vi "AlliGator Run Source Image Python Function.vi"(8 "error in (no error)":errorcluster, 9 "Source Image":T5, 10 "Python Function Info":T1={"Script Path"=path "", "Function Name"="", "Function Parent Menu"="", "API Version"="", "Function Input Parameters"=[], "Function Outputs"=[], "Function Doc String"="", "Function Display Name"="", "Function Target Type"=enum."Window Menu", "Function Target Window"="", "Parent Menu Location"="", "Item Menu Tag"="", "Is preceded by Separator"=FALSE}, 11 "Data Value Reference in":refnum<data-value>) -> (0 "error out":errorcluster, 1 "Message":string, 2 "Function Output Type":string, 3 "Data Value Reference out":refnum<data-value>)   [LabVIEW 2021, in "AlliGator Python Plugins.lvlib"]
doc: "Runs image-related python function."
uses:
  AlliGator Python Plugins.lvlib
  Internal Variables/AlliGator Internal Variables v2.ctl
  <vilib>/vision/Image Controls.llb/IMAQ Image.ctl
  Internal Variables/AlliGator Gate Image Set.ctl
  Files/AlliGator FLI Dataset Type.ctl
  Files/AlliGator Data Series Type.ctl
  Dual-Channel Datasets/AlliGator Dataset Channel.ctl
  Settings/AlliGator Gate Arithmetic.ctl
  Source Image/AlliGator Displayed Image.ctl
  Image/Named ROI Description.ctl
  Phasor Graph/AlliGator Decay Metadata v3.ctl
  Decay Analysis/Decay Preprocessing/AlliGator Decay Background Subtraction Info.ctl
  Decay Analysis/Decay Preprocessing/AlliGator Baseline Subtraction Method.ctl
  Graphs/XY Graph/XY Graph Plot Shift Parameters.ctl
  Graphs/XY Graph/XY Graph Plot Shift Method.ctl
  Decay Analysis/Decay Preprocessing/AlliGator Decay Extrapolation Parameters.ctl
  Phasor/Calibration Phasor (m, phi).ctl
  Phasor/Phasor Reference Series.ctl
  Phasor/Phasor Calibration Map v2.ctl
  Phasor/Phasor (g, s).ctl
  Phasor Graph/AlliGator Raw Phasor Plot Data v5.ctl
  Phasor/Phasor Standard Deviation Options.ctl
  Phasor Plot/AlliGator Phasor Multi-Harmonic Data.ctl
  Phasor/Phasor Harmonic Data.ctl
  Decay Fit Parameter Map/AlliGator Decay Fit Options & Parameters v4.ctl
  Fits/IRF(X)PSED/Decay Fit Options v4.ctl
  Fits/Decay Convolution/Decay Model.ctl
  Fits/Residual Type.ctl
  Fits/IRF(X)PSED/Fit Weights Type v2.ctl
  Fits/Non-linear Fitting Method v2.ctl
  Fits/Fit Calculation Method.ctl
  Fits/Non-linear Fitting Algorithm.ctl
  Decay Analysis/Decay Fit/AlliGator Decay Fit Parameter Constraints 2.ctl
  Fits/IRF(X)PSED/Decay Fit Parameters In List.ctl
  Fits/IRF(X)PSED/MLE Baseline Offset Type.ctl
  Decay Analysis/Decay Preprocessing/AlliGator Decay Preprocessing Parameters.ctl
  Fits/IRF(X)PSED/Decay Fit Parameters & Derived Quantities List v2.ctl
  Fits/IRF(X)PSED/Decay Fit Result Constraint.ctl
  Decay Fit Parameter Map/AlliGator Parameter Maps Data.ctl
  AlliGator Python Function Information.ctl
  AlliGator Python Function Parameter Definition.ctl
  AlliGator Python Function Output Definition.ctl
  AlliGator Python Plugin Target Type.ctl
  Globals, Variables, Constants/AlliGator Variables List.ctl
  API v1/AlliGator Python Plugin Image Data v1.ctl
  API v1.1/AlliGator Python Plugin Data v1.1.ctl
  API v1/AlliGator Python Plugin Graph Data v1.ctl
  API v1/AlliGator Python Plugin Plot Data v1.ctl
  API v1.1/AlliGator Python Plugin Parameter Map Data v1.1.ctl
  Image/Image Point.ctl
  API v1.1/AlliGator Python Plugin FLI Dataset Data v1.1.ctl
  Globals, Variables, Constants/AlliGator Globals, Variables & Constants.lvlib
  Source Image/AlliGator Source Image.lvlib
  Error/Error.lvlib
  Strings/Strings.lvlib
  Image/Image.lvlib
  Phasor/Phasor.lvlib
  Decay Analysis/Decay Preprocessing/AlliGator Decay Preprocessing.lvlib
  Graphs/XY Graph/XY Graph Add-Ons.lvlib
  Phasor Graph/AlliGator Phasor Graph.lvlib
  Files/AlliGator Files.lvlib
  Phasor Plot/AlliGator Phasor Plot.lvlib
  Fits/Fits.lvlib
  Decay Analysis/Decay Fit/AlliGator Decay Fit.lvlib
  Internal Variables/AlliGator Internal Variables.lvlib
  Settings/AlliGator Settings.lvlib
  Dual-Channel Datasets/AlliGator Dual-Channel Datasets.lvlib
  Decay Fit Parameter Map/AlliGator Decay Fit Parameter Map.lvlib
panel:
  out "session out":refnum<k35>
  out "Function Parameters String":string
  # "see the AlliGator License on the block diagram (Ctrl+E or Window:Show Block Diagram)"
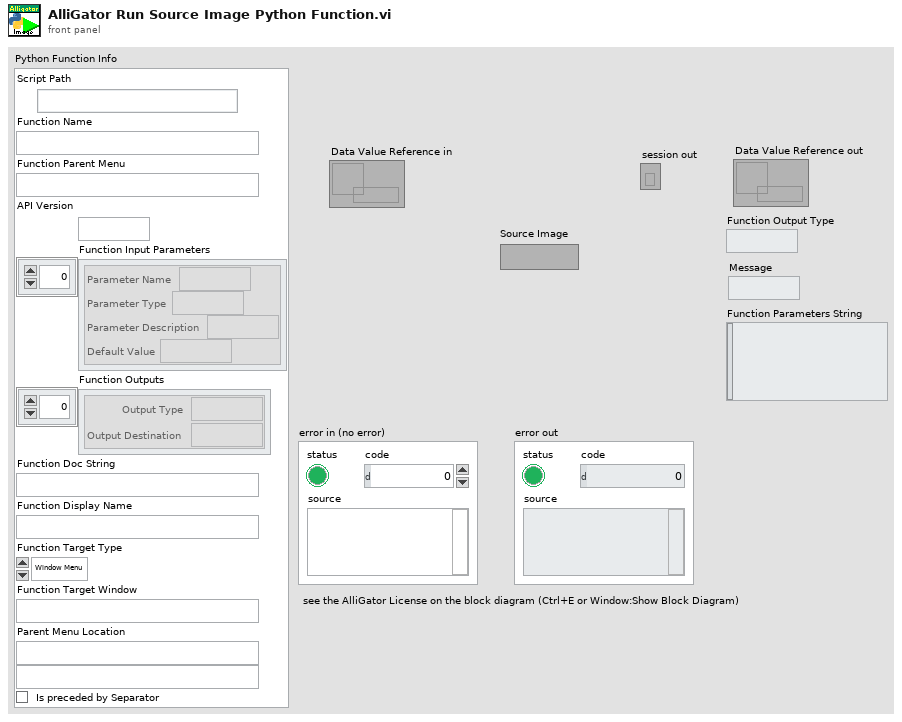
[diagram p1: front panel]
types:
  T1 = typedef "AlliGator Python Plugins.lvlib/AlliGator Python Function Information.ctl" = cluster{"Script Path":path, "Function Name":string, "Function Parent Menu":string, "API Version":string, "Function Input Parameters":T2[], "Function Outputs":T3[], "Function Doc String":string, "Function Display Name":string, "Function Target Type":T4, "Function Target Window":string, "Parent Menu Location":string, "Item Menu Tag":string, "Is preceded by Separator":bool}
  T2 = typedef "AlliGator Python Plugins.lvlib/AlliGator Python Function Parameter Definition.ctl" = cluster{"Parameter Name":string, "Parameter Type":string, "Parameter Description":string, "Default Value":string}
  T3 = typedef "AlliGator Python Plugins.lvlib/AlliGator Python Function Output Definition.ctl" = cluster{"Output Type":string, "Output Destination":string}
  T4 = typedef "AlliGator Python Plugins.lvlib/AlliGator Python Plugin Target Type.ctl" = enum16{"Undefined", "Window Menu", "Object Menu"}
  T5 = typedef "IMAQ Image.ctl" = refnum<image>
  T6 = typedef "AlliGator Python Plugins.lvlib/AlliGator Python Plugin Data v1.1.ctl" = cluster{"Image_Plugin_Data":T7, "Graph_Plugin_Data":T8, "Parameter_Map_Plugin_Data":T10, "FLI_Dataset_Plugin_Data":T12}
  T7 = typedef "AlliGator Python Plugins.lvlib/AlliGator Python Plugin Image Data v1.ctl" = cluster{"Image_Name":string, "Image":sgl[][]}
  T8 = typedef "AlliGator Python Plugins.lvlib/AlliGator Python Plugin Graph Data v1.ctl" = cluster{"Graph_Name":string, "Plots":T9[], "Reference_Decay":T9}
  T9 = typedef "AlliGator Python Plugins.lvlib/AlliGator Python Plugin Plot Data v1.ctl" = cluster{"Plot_Name":string, "X_Array":dbl[], "Y_Array":dbl[]}
  T10 = typedef "AlliGator Python Plugins.lvlib/AlliGator Python Plugin Parameter Map Data v1.1.ctl" = cluster{"Parameter_Names":string[], "Parameter_Flattened_Map":dbl[][], "Locations":T11[], "IRF_X":dbl[], "IRF_Y_Flattened_List":dbl[][], "X_Resolution":i32, "Y_Resolution":i32}
  T11 = typedef "Image.lvlib/Image Point.ctl" = cluster{"X":i32, "Y":i32}
  T12 = typedef "AlliGator Python Plugins.lvlib/AlliGator Python Plugin FLI Dataset Data v1.1.ctl" = cluster{"FLI_Dataset_Name":string, "Gate_Duration":dbl, "Gate_Separation":dbl, "Gate_Number":i32, "X_Size":i32, "Y_Size":i32, "Image_Data_List":T7[], "Mask_Image":u16[][], "Sum_Image":sgl[][], "Max_Image":sgl[][], "Min_Image":sgl[][]}
  T13 = typedef "AlliGator Source Image.lvlib/AlliGator Displayed Image.ctl" = enum16{"Single Gate", "Sum of All Gates", "Max of All Gates", "Min of All Gates", "-", "White Ligth Image", "Mask Image"}
  T14 = typedef "AlliGator Globals, Variables & Constants.lvlib/AlliGator Variables List.ctl" = enum16{"---- GUI ----", "GUI:Initialization Status", "GUI:State Indicators Refnum", "GUI:Original AlliGator Menu Items", "GUI:Current Action Loop State", "GUI:Script in progress", "GUI:Playback", "GUI:Loop Playback", "GUI:Search ROI Used", "GUI:Search ROI", "Decay Graph Max Legend Size", "Intensity Graph Max Legend Size", "Decay Statistics Graph Max Legend Size", "Phasor Graph Max Legend Size", "Phasor Ratio Graph Max Legend Size", "Lifetime Graph Max Legend Size", "---- Files ----", "Files:Export Dataset Frames as Individual Files", "Files:Show Batch Export Help Balloons", "Files:Frames in Dataset", "Files:ptu File Frame Start Indices", "Files:Current Frame in Dataset", "Files:Current Frame Timestamp", "Files:Dataset Loaded", "Files:Dataset Metadata", "Files:Dataset Channel", "Files:Dataset Data Description", "Files:Background Dataset Metadata", "Files:Background Dataset Channel", "Files:Background Dataset Data Description", "Files:Background File Subtraction", "Files:Background File Path", "Files:Background File Pile-up Correction", "Files:Background File Pixel Well Capacity", "Files:Background File Scaling Factor", "Files:Current Dataset Load Settings", "Files:Dataset Path", "Files:ICCD-specific Information", "Files:Macrotime Gate Separation", "------ Python Plugins ------", "Python Plugins:Information", "Python Plugins:Python Session", "Python Plugins:Valid Python Session?", "---- Source Image ----", "Source Image:ROIs", "Source Image:Current ROI", "Source Image:ROI Event Refnum", "X_Source Image:Display Range", "X_Source Image:Palette Information", "X_Source Image:Type of Displayed Image", "X_Time Gate Slider", "Source Image:Palette List", "Source Image:Scale", "Source Image:ROI Overlay Color", "Source Image:Overlay to Erase", "Source Image:Is Displayed Image Accumulated", "Source Image:White Light Image Modified", "Source Image:Mask Image Modified", "---- Image Profile Window ----", "Image Profile:Window Event Refnum", "Image Profile:IntensityType", "Image Profile:Intensity Average Type", "Image Profile:Intensity-weighted SDV", "Image Profile:Box Profile Type", "Image Profile:Window Open", "Image Profile:Plotted Fit Parameter", "------ Phasor Graph -------", "Phasor Graph:Show Line", "---- Phasor Plot ---", "Phasor Plot:Parameters Changed", "Phasor Plot:FLI Dataset Modified since last Calculation", "Phasor Harmonics Data", "Selected Phasor Harmonics", "Phasor Harmonic Manager Event Refnum", "Phasor Plot:ROIs", "Phasor Plot:Current ROI", "Phasor Plot:ROI Event Refnum", "Phasor Plot:Image Reference Points", "Phasor Plot:Computed", "Phasor Plot:Palette Information", "Phasor Plot:Palette List", "Phasor Plot:Phasor Ratio Palette Information", "Phasor Plot:Phasor Ratio Palette List", "Phasor Plot:Image Scale", "Phasor Plot:Image Overlay to Erase", "Phasor Plot:Image Elements to Update", "Phasor Plot:Current Calculation Parameters", "Phasor Plot:Current Calibration Options", "Phasor Plot:Reset Cumulated Phasor Plot", "Phasor Plot:Reference 1", "Phasor Plot:Lifetime Reference 1", "Phasor Plot:Reference 1 Frequency", "Phasor Plot:Reference 2", "Phasor Plot:Lifetime Reference 2", "Phasor Plot:Reference 2 Frequency", "---- Decay Analysis ----", "Number of Selected Decays to Fit", "LS Fit Results", "LAR Fit Results", "BS Fit Results", "Last Decay Max - Min", "Best Fit Parameters", "Best Fit Parameter Names", "Actual Size X", "Actual Size Y", "Binning X", "Binning Y", "Actual # Gates", "Dataset Number", "Gates to...", "Gates Skipped", "Gates to keep", "Gate Step", "Gate Separation", "Reversed Gates", "Pile-up Correction", "Pixel Well Capacity", "Background Subtracted", "Background Subtraction Method", "Background Definition Range", "Background File (deprecated)", "Number of Dataset Accumulated", "Array of Accumulated Dataset Paths", "Do Averaged Datasets", "Destination File Path", "Process Plot Target", "Use 1/D as Phasor Frequency", "---- Decay Fit Parameter Map -----", "Decay Fit Parameter Map:Palette Information", "Decay Fit Parameter Map:Palette List", "Decay Fit Parameter Map:X Resolution", "Decay Fit Parameter Map:Y Resolution", "Decay Fit Parameter Map:Use Decay Fit Result Constraints", "Decay Fit Parameter Map:Decay Fit Result Constraints", "Decay Fit Parameter Map:Decay Fit Result Constraints Applied", "---- Parameter Map ----", "Parameter Map:Palette Information", "Parameter Map:Palette List", "------- Local Decay Window ---------", "Local Decay Graph Window:Event Refnum", "Local Decay Graph Window:Use normalized IRF for convolution", "----- Miscellaneous ----", "Misc:Skippable Dialog Windows Status"}
  T15 = typedef "AlliGator Internal Variables.lvlib/AlliGator Internal Variables v2.ctl" = cluster{"----------------------------- Images -----------------------------":u8, "Displayed Image":T5, "White Light Image":T5, "Mask Image":T5, "ROI Mask Image":T5, "Current Dataset Images 1":T16, "Background Dataset Images 1":T16, "Current Dataset Images 2":T16, "Background Dataset Images 2":T16, "Current Dataset Arithmetic Images":T16, "Accumulated Dataset Images 1":T16, "Accumulated Dataset Images 2":T16, "Accumulated Dataset Arithmetic Images":T16, "----------------------------- File Paths -----------------------------":u8, "Phasor Plot Image":T5, "Decay Fit Parameter Map Image":T5, "Parameter Map Image":T5, "Single Data Point Path":path, "White Light Image Path":path, "Mask Image Path":path, "Time-Series Folder":path, "[Time-Series Paths]":path[], "----------------------------- FLI Dataset -----------------------------":u8, "Current Dataset":i32, "Single Dataset Type":T17, "Current Folder":string, "AlliGator Data Series Type":T18, "# Datasets":i32, "Dual-Channel Dataset":bool, "Selected Channel Name":string, "Dataset Channel":T19, "Channel Arithmetic":T20, "Dual-Channel Background Dataset":bool, "Background Channel":T19, "Dual-Channel Accumulated Dataset":bool, "Start Time":dbl, "[Time-Series Timestamps]":dbl[], "[Intensity Corrections]":dbl[], "Time Series Script":bool, "Type of Displayed Image":T13, "Gate Image Slide":u16, "# Gates":i32, "ROIs":T21[], "----------------------------- Decays -----------------------------":u8, "ROI Decay":cluster{"t Array":dbl[], "I Array":dbl[]}, "Valid Decay":bool, "Decay  Metadata":T23, "Reference Decay Plot Name":string, "Reference Decay":cluster{"t Array":dbl[], "I Array":dbl[]}, "Decay Shift Plot":cluster{"Time Stamps":dbl[], "Decay Shifts":dbl[]}, "[Decays Max Values]":sgl[], "[Decays Min Values]":sgl[], "----------------------------- Calibration -----------------------------":u8, "Calibration Phasor":T29, "Calibration Phasor Series":T30, "Phasor Calibration Map":T31, "Calibration Map MD5 Digest":string, "----------------------------- Phasor Graph -----------------------------":u8, "Last Raw Phasor":T32, "Last Calibrated Phasor":T32, "Last Calibrated Phasor SDV":T32, "Phasor Graph:Phasor Plot":cluster{"g Array":dbl[], "s Array":dbl[]}, "Phasor Graph:Phasor SDV Plot":cluster{"g Array":dbl[], "s Array":dbl[]}, "[Phasor Graph:Raw Phasor Plots]":T33[], "Phasor Plot locked to Ref 1":i32, "[Phasor Plot(s) locked to Ref 1]":i32[], "[Phasor Plot(s) locked to Ref 2]":i32[], "[Pixel Phasors]":T32[], "----------------------------- Phasor Plot -----------------------------":u8, "[[Sum Image]]":dbl[][], "[[CSG Phasors]]":csg[][], "[[Valid Pixel?]]":bool[][], "[[Phasor Ratios]]":dbl[][], "[[Average Lifetimes]]":dbl[][], "Amplitude Weighted Average Lifetime":bool, "I/m/phi Dataset":cluster{"I/m/phi Dataset?":bool, "Base Frequency":dbl[unit], "Harmonic Orders":u8[]}, "Multi Phasor Plot Data":T35, "----------------------------- Decay Fit Parameter Map -----------------------------":u8, "Decay Fit Options & Parameters":T37, "Fit Options: Decay Preprocessing Parameters":T48, "Fit Options: Reference Decay":cluster{"t Array":dbl[], "I Array":dbl[]}, "Is Full Image Parameters Map":bool, "Is Single-Pixels Parameters Map":bool, "NLSF Parameters Map X Resolution":i32, "NLSF Parameters Map Y Resolution":i32, "[Single Decay Fit Parameters]":dbl[], "Fit Model":T39, "[[Multiple Decays Fit Parameters]]":dbl[][], "[[Multiple Decays Fit Parameter SDVs]]":dbl[][], "[[IRFs]]":dbl[][], "[ROI Descriptors]":T22[], "IRF Array Time Axis":dbl[], "Decay Array Time Axis":dbl[], "[Decay Fit Parameter Names]":T49[], "[Decay Sum]":dbl[], "Array of Decay Fit Result Constraints":T50[], "Selected ROIs Array":bool[], "----------------------------- Parameter Maps -----------------------------":u8, "[Map Set Names]":string[], "[Parameter Maps]":T51[], "[[User-defined Quantities]]":dbl[][], "User-defined Quantity":string}
  T16 = typedef "AlliGator Internal Variables.lvlib/AlliGator Gate Image Set.ctl" = cluster{"SGL Gate Images":T5[], "SGL Sum Image":T5, "SGL Max Image":T5, "SGL Min Image":T5}
  T17 = typedef "AlliGator Files.lvlib/AlliGator FLI Dataset Type.ctl" = enum16{"HDF5 FLI Dataset", "Gate Image Folder", ".sdt FLI Dataset (Becker & Hickl)", ".ptu FLI Dataset (PicoQuant)", "SS1 FLI Dataset", "SS2 FLI Dataset", "I/m/phi Dataset", ".bin FLI Dataset (PicoQuant Binned)", ".bin FLI Dataset (Piccolo Binned)", ".mat FLI Dataset"}
  T18 = typedef "AlliGator Files.lvlib/AlliGator Data Series Type.ctl" = enum16{"Not a Supported Series", "Gate Images Folder Series", "SwissSPAD 2 Dataset Series", "B&H FLI Dataset Series", "PicoQuant PTU FLI Dataset Series", "PicoQuant BIN FLI Dataset Series", "Piccolo hist BIN FLI Dataset Series", "HDF5 FLI Dataset Series"}
  T19 = typedef "AlliGator Dual-Channel Datasets.lvlib/AlliGator Dataset Channel.ctl" = enum16{"G2", "INT"}
  T20 = typedef "AlliGator Settings.lvlib/AlliGator Gate Arithmetic.ctl" = enum16{"None", "INT-G2", "G2/INT*<INT>", "(1 - G2/INT)*<INT>"}
  T21 = typedef "Image.lvlib/Named ROI Description.ctl" = cluster{"ROI Descriptor":T22, "ROI Name":string, "Overlay Color":u32}
  T22 = typedef "ROI Descriptor" = cluster{"Global Rectangle":i32[], "Contours":cluster{"ID":enum32{"External", "Internal"}, "Type":u32, "Coordinates":i32[]}[]}
  T23 = typedef "AlliGator Phasor Graph.lvlib/AlliGator Decay Metadata v3.ctl" = cluster{"ROI Descriptor":T22, "ROI Center":cluster{"X":i32, "Y":i32}, "Decay Background Subtraction Info":T24, "Decay Reverted":bool, "Decay Smoothened":bool, "Decay Straightened":bool, "Fitted Tau (Decay Straightening)":dbl, "Decay Shift Parameters":T26, "Decay Shifted":bool, "Decay Extrapolated":bool, "Decay Extrapolation Parameters":T28, "Decay Normalized":bool, "Fold Decay":bool, "# Folds":u32}
  T24 = typedef "AlliGator Decay Preprocessing.lvlib/AlliGator Decay Background Subtraction Info.ctl" = cluster{"Laser Period":dbl[unit], "Gate Duration":dbl[unit], "Baseline Subtraction Method":T25, "Background Definition Range":cluster{"Min Gate":dbl[unit], "Max Gate":dbl[unit]}, "Total Intensity w/o Bkgd Subtraction":dbl, "Bkgd-subtracted Intensity (exp)":dbl, "# Data Points":i32, "Background/Gate":dbl, "Fitted Lifetime":dbl[unit], "Bkgd-subtracted Intensity (theo)":dbl}
  T25 = typedef "AlliGator Decay Preprocessing.lvlib/AlliGator Baseline Subtraction Method.ctl" = enum16{"Mean", "Min", "Square Gated Single-Exponential", "File", "Constant"}
  T26 = typedef "XY Graph Add-Ons.lvlib/XY Graph Plot Shift Parameters.ctl" = cluster{"Type":T27, "Shift":dbl[unit], "Threshold":dbl, "Rotate":bool}
  T27 = typedef "XY Graph Add-Ons.lvlib/XY Graph Plot Shift Method.ctl" = enum16{"Default", "CFD", "Threshold", "Cross-Correlation"}
  T28 = typedef "AlliGator Decay Preprocessing.lvlib/AlliGator Decay Extrapolation Parameters.ctl" = cluster{"Additional Points":u32, "Head Fraction":dbl, "Fitted Tau":dbl, "Use Periodicity":bool, "Use Cursors":bool, "Tail Fraction":dbl}
  T29 = typedef "Phasor.lvlib/Calibration Phasor (m, phi).ctl" = cluster{"m":dbl, "phi":dbl, "Phasor Frequency":dbl[unit], "Reference Lifetime":dbl[unit]}
  T30 = typedef "Phasor.lvlib/Phasor Reference Series.ctl" = cluster{"m Array":dbl[], "phi Array":dbl[], "Phasor Frequency":dbl[unit], "Calibration Lifetime":dbl[unit]}
  T31 = typedef "Phasor.lvlib/Phasor Calibration Map v2.ctl" = cluster{"Phasor Frequency":dbl[unit], "Calibration Lifetime":dbl[unit], "ROI Centers":cluster{"X":i32, "Y":i32}[], "ROI Descriptors":T22[], "Map Resolution X":i32, "Map Resolution Y":i32, "z Array":cdb[]}
  T32 = typedef "Phasor.lvlib/Phasor (g, s).ctl" = cluster{"g":dbl, "s":dbl}
  T33 = typedef "AlliGator Phasor Graph.lvlib/AlliGator Raw Phasor Plot Data v5.ctl" = cluster{"Phasor Plot Name":string, "Raw Phasor Plot":T32[], "Phasor Frequency":dbl[unit], "[Decay Metadata]":T23[], "Raw Phasor Plot SDV":T32[], "Phasor SDV Options":T34, "[Calibration Phasor]":T29[], "Intensity Array":dbl[]}
  T34 = typedef "Phasor.lvlib/Phasor Standard Deviation Options.ctl" = cluster{"Compute Estimated SDV":bool, "# Replicas":u32, "Use Estimated Average Phasor":bool}
  T35 = typedef "AlliGator Phasor Plot.lvlib/AlliGator Phasor Multi-Harmonic Data.ctl" = cluster{"Base Frequency":dbl[unit], "# Harmonics":u8, "Harmonic Orders":u8[], "Phasor Plot Settings Checksum":u64, "Phasor Harmonic Data Array":T36[]}
  T36 = typedef "Phasor.lvlib/Phasor Harmonic Data.ctl" = cluster{"Phasor Harmonic Name":string, "Phasor Plot Settings Checksum":u64, "Phasor Frequency":dbl[unit], "Base Frequency":dbl[unit], "Harmonic Order":u8, "Phasor Plot Parameters":string, "Phasor Array [[CSG]]":csg[][], "Dataset File Path":path}
  T37 = typedef "AlliGator Decay Fit Parameter Map.lvlib/AlliGator Decay Fit Options & Parameters v4.ctl" = cluster{"SYNC Period":dbl[unit], "Fit Options":T38, "Fit Parameter Constraints":T45[], "MLE Baseline Offset":dbl, "MLE Baseline Offset Type":T47}
  T38 = typedef "Fits.lvlib/Decay Fit Options v4.ctl" = cluster{"Show Fit Residuals":bool, "Fit Model":T39, "Residual Type":T40, "Max Decay Percentile":dbl, "Min Decay Percentile":dbl, "Show Full Decay":bool, "Weights":T41, "Fitting Method":T42, "Compute Parameter Uncertainties":bool, "Periodic Boundaries":bool, "Model Calculation":T43, "Period":dbl[unit], "Termination Criteria":cluster{"Max Iterations":i32, "Max Function Calls":i32, "Max Time":dbl[unit], "Function Tolerance":dbl, "Parameter Tolerance":dbl, "Gradient Tolerance":dbl, "Min Lambda":dbl, "Max Lambda":dbl, "Initial Tick Count":u32}, "Offset Resolution":dbl[unit], "Use Local IRF":bool, "Fitting Algorithm":T44, "Show Confidence Interval ":bool, "Confidence Level":dbl}
  T39 = typedef "Fits.lvlib/Decay Model.ctl" = enum16{"1-Exponential", "2-Exponentials"}
  T40 = typedef "Fits.lvlib/Residual Type.ctl" = enum16{"Standard", "Normalized", "Reduced"}
  T41 = typedef "Fits.lvlib/Fit Weights Type v2.ctl" = enum16{"Unweighted", "1/Variance (Neyman)", "1/Variance (Pearson)", "Best of All"}
  T42 = typedef "Fits.lvlib/Non-linear Fitting Method v2.ctl" = enum16{"Least Square", "Least Absolute Residual", "Bisquare", "MLE", "-", "Best of All"}
  T43 = typedef "Fits.lvlib/Fit Calculation Method.ctl" = enum16{"Simulation", "Convolution", "Integration"}
  T44 = typedef "Fits.lvlib/Non-linear Fitting Algorithm.ctl" = enum16{"Levenberg-Marquardt", "Trust-Region Dogleg"}
  T45 = typedef "AlliGator Decay Fit.lvlib/AlliGator Decay Fit Parameter Constraints 2.ctl" = cluster{"Fit Parameter":T46, "Min Value":dbl, "Max Value":dbl, "Global":bool, "Used":bool}
  T46 = typedef "Fits.lvlib/Decay Fit Parameters In List.ctl" = enum16{"Offset", "Baseline", "A_1", "tau_1", "A_2", "tau_2"}
  T47 = typedef "Fits.lvlib/MLE Baseline Offset Type.ctl" = enum32{"Absolute", "Percentage"}
  T48 = typedef "AlliGator Decay Preprocessing.lvlib/AlliGator Decay Preprocessing Parameters.ctl" = cluster{"Background Subtraction":bool, "Straighten Decay":bool, "Reverse Gates":bool, "1-Normalized Decay":bool, "Smoothen Decay":bool, "Smoothing Parameter":dbl, "Shift Decay":bool, "Decay Shift Parameters":T26, "Extrapolate Decay":bool, "Additional Points":u32, "Head Fraction":dbl, "Pixel-Normalize Decay":bool, "Use Periodicity":bool, "Use Cursors":bool, "Tail Fraction":dbl, "Use Decay Pre-Processing":bool, "Fold Decay":bool, "# Folds":u32, "[0-1]-Normalized Decay":bool}
  T49 = typedef "Fits.lvlib/Decay Fit Parameters & Derived Quantities List v2.ctl" = enum16{"Offset", "Baseline", "A_1", "tau_1", "A_2", "tau_2", "<tau>_a", "f1_a", "f2_a", "<tau>_i", "f1_i", "f2_i", "-", "R^2", "Chi^2"}
  T50 = typedef "Fits.lvlib/Decay Fit Result Constraint.ctl" = cluster{"Fit Parameter":enum16{"Offset", "Baseline", "A_1", "tau_1", "A_2", "tau_2", "<tau>_a", "f1_a", "f2_a", "<tau>_i", "f1_i", "f2_i", "-", "R^2", "Chi^2", "Max Relative Residual", "<Residual ACF>", "Residual ACF SDV", "tau_2/tau_1"}, "Min Value":dbl, "Max Value":dbl, "Use Constraint":bool}
  T51 = typedef "AlliGator Decay Fit Parameter Map.lvlib/AlliGator Parameter Maps Data.ctl" = cluster{"Map Set Name":string, "[Parameter Names]":string[], "[[Parameters]]":dbl[][], "[[Parameter SDVs]]":dbl[][], "Decay Array Time Axis":dbl[], "[[IRFs]]":dbl[][], "IRF Array Time Axis":dbl[], "X Resolution":i32, "Y Resolution":i32, "Intensity Array":dbl[]}
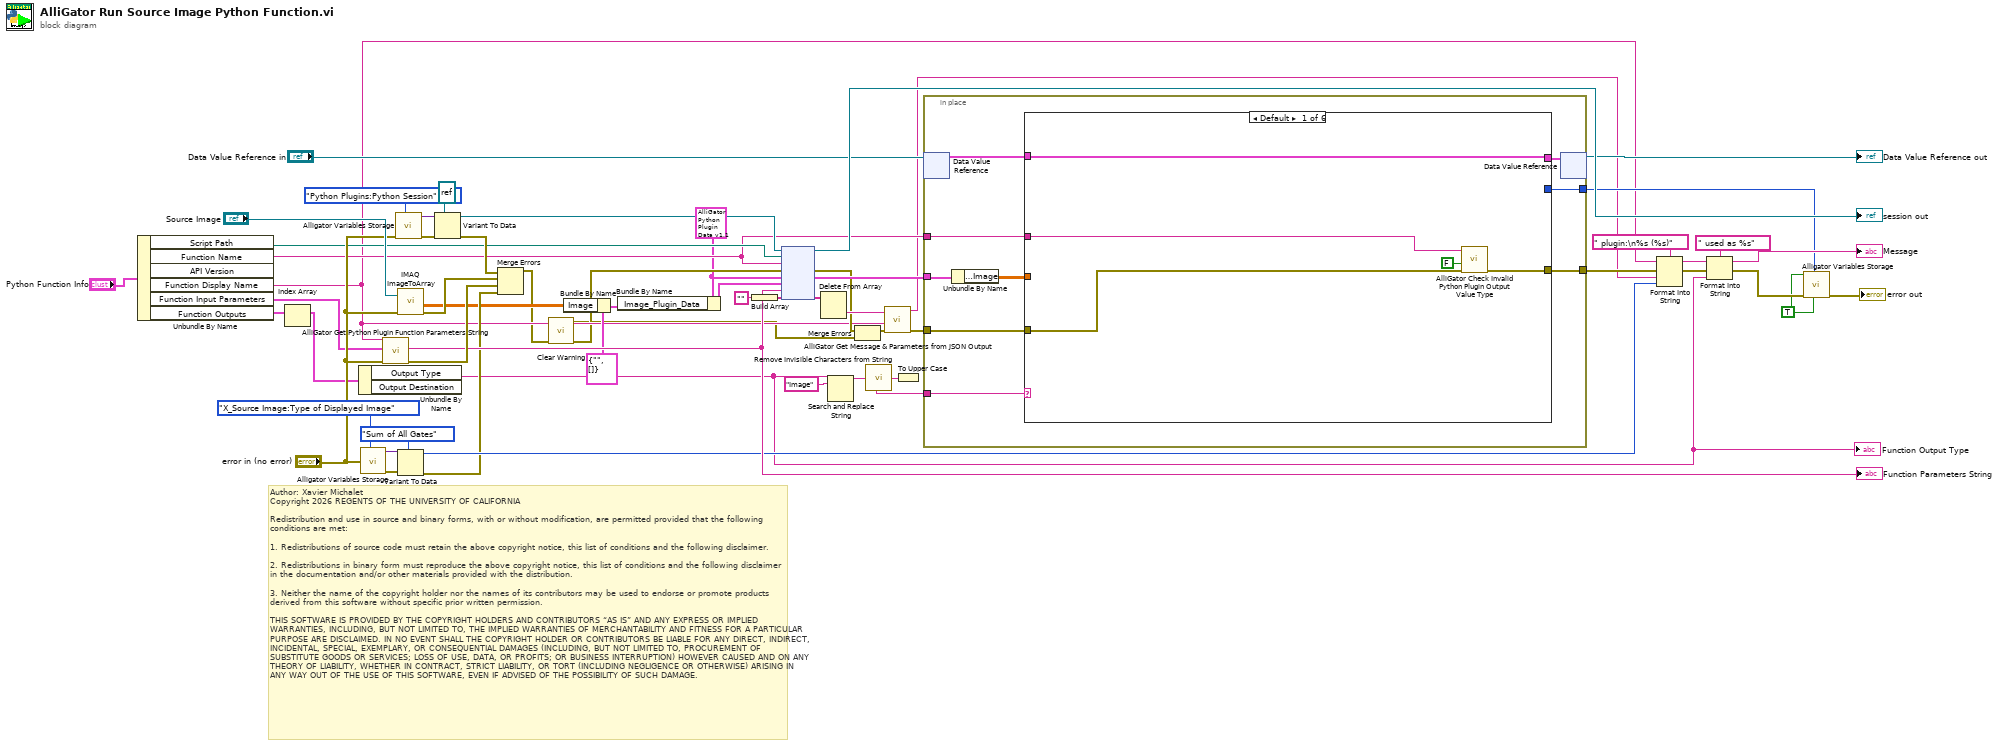
[diagram p0: block diagram]
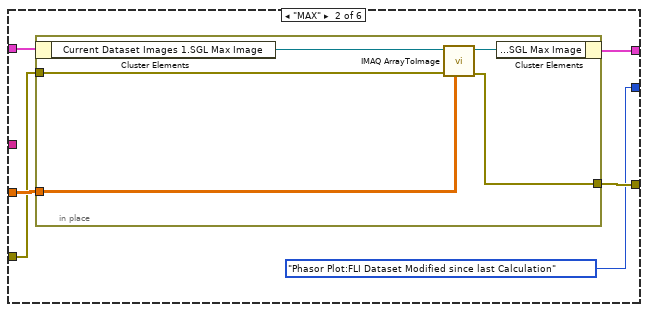
[diagram p2: hidden frame]
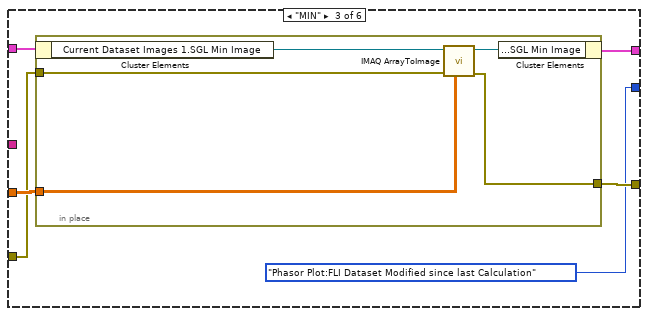
[diagram p3: hidden frame]
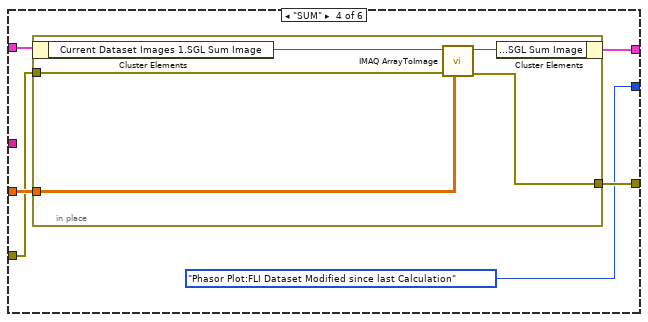
[diagram p4: hidden frame]
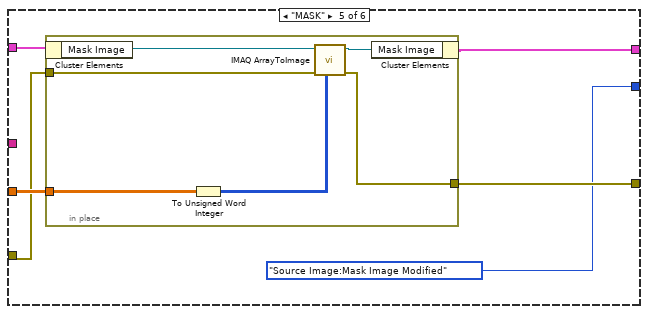
[diagram p5: hidden frame]
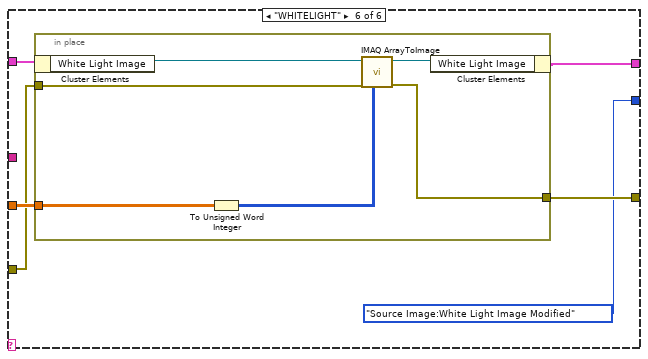
[diagram p6: hidden frame]
diagram:
  w1 = T6 {"Image_Plugin_Data"={"Image_Name"="", "Image"=[]}, "Graph_Plugin_Data"={"Graph_Name"="", "Plots"=[], "Reference_Decay"={"Plot_Name"="", "X_Array"=[], "Y_Array"=[]}}, "Parameter_Map_Plugin_Data"={"Parameter_Names"=[], "Parameter_Flattened_Map"=[], "Locations"=[], "IRF_X"=[], "IRF_Y_Flattened_List"=[], "X_Resolution"=0, "Y_Resolution"=0}, "FLI_Dataset_Plugin_Data"={"FLI_Dataset_Name"="", "Gate_Duration"=0.0, "Gate_Separation"=0.0, "Gate_Number"=0, "X_Size"=0, "Y_Size"=0, "Image_Data_List"=[], "Mask_Image"=[], "Sum_Image"=[], "Max_Image"=[], "Min_Image"=[]}} ("Plugin_Data")
  w35 = TRUE ("Get(F)/Set")
  # "Author: Xavier Michalet\nCopyright 2026 REGENTS OF THE UNIVERSITY OF CALIFORNIA\n\nRedistribution and use in source and binary forms, with or without modification, are permitted provided that the following conditions are met:\n\n1. Redistributions of source code must retain the above copyright notice, this list of conditions and the following disclaimer.\n\n2. Redistributions in binary form must reproduce the above copyright notice, this list of conditions and the following disclaimer in the documentation and/or other materials provided with the distribution.\n\n3. Neither the name of the copyright holder nor the names of its contributors may be used to endorse or promote products derived from this software without specific prior written permission.\n\nTHIS SOFTWARE IS PROVIDED BY THE COPYRIGHT HOLDERS AND CONTRIBUTORS “AS IS” AND ANY EXPRESS OR IMPLIED WARRANTIES, INCLUDING, BUT NOT LIMITED TO, THE IMPLIED WARRANTIES OF MERCHANTABILITY AND FITNESS FOR A PARTICULAR PURPOSE ARE DISCLAIMED. IN NO EVENT SHALL THE COPYRIGHT HOLDER OR CONTRIBUTORS BE LIABLE FOR ANY DIRECT, INDIRECT, INCIDENTAL, SPECIAL, EXEMPLARY, OR CONSEQUENTIAL DAMAGES (INCLUDING, BUT NOT LIMITED TO, PROCUREMENT OF SUBSTITUTE GOODS OR SERVICES; LOSS OF USE, DATA, OR PROFITS; OR BUSINESS INTERRUPTION) HOWEVER CAUSED AND ON ANY THEORY OF LIABILITY, WHETHER IN CONTRACT, STRICT LIABILITY, OR TORT (INCLUDING NEGLIGENCE OR OTHERWISE) ARISING IN ANY WAY OUT OF THE USE OF THIS SOFTWARE, EVEN IF ADVISED OF THE POSSIBILITY OF SUCH DAMAGE."
  n1 = Unbundle By Name("Python Function Info") -> ("Script Path"=w30:path, "Function Name"=w21:string, "Function Display Name"=w11:string, "Function Input Parameters"=w29:T2[], "Function Outputs"=w26:T3[])  [unwired: 1 out]
  n2 = Index Array(array=w26) -> (element=w25:T3)  [unwired: 1 in]
  n3 = Unbundle By Name(w25) -> ("Output Type"=w24:string)  [unwired: 1 out]
  "Function Output Type" <- w24
  n4 = call "Alligator Variables Storage.vi"("AlliGator Variable"=AlliGator_Variables_List."X_Source Image:Type of Displayed Image" ("Alligator Variable"), "Error In"="error in (no error)") -> ("Error Out"=w44:errorcluster, "Data out"=w45:variant)  [unwired: 7 in, 1 out]
  n5 = call "AlliGator Get Python Plugin Function Parameters String.vi"("error in (no error)"="error in (no error)", "Function Parameters"=w29, "Function Display Name"=w11) -> ("error out"=w57:errorcluster, "Function Parameters JSON String"=w56:string)  [unwired: 6 in, 1 out]
  "Function Parameters String" <- w56
  n6 = call "Alligator Variables Storage.vi"("AlliGator Variable"=AlliGator_Variables_List."Python Plugins:Python Session" ("Alligator Variable"), "Error In"="error in (no error)") -> ("Error Out"=w54:errorcluster, "Data out"=w52:variant)  [unwired: 7 in, 1 out]
  n7 = call "IMAQ ImageToArray"("error in (no error)"="error in (no error)", "Image"="Source Image") -> ("Image Pixels (Float)"=w13:sgl[][], "error out"=w32:errorcluster)  [unwired: 2 in, 3 out]
  n8 = Variant To Data(error in=w44, type=AlliGator_Displayed_Image."Sum of All Gates" ("Displayed Image"), Variant=w45) -> (data=w42:T13, error out=w41:errorcluster)
  n9 = Variant To Data(error in=w54, type=refnum<k35> refnum ("session in"), Variant=w52) -> (data=w50:refnum<k35>, error out=w53:errorcluster)
  n10 = Merge Errors(w53, w32, w57, w41) -> (w10:errorcluster)
  n11 = call "Clear Warning.vi"("error in (no error)"=w10) -> ("cleared warning or error dup"=w9:errorcluster, "error in (dup)"=w7:errorcluster)  [unwired: 9 in]
  n12 = Bundle By Name(cluster=T7 {"Image_Name"="", "Image"=[]} ("Image_Data"), "Image"=w13) -> (w3:T7)
  n13 = Bundle By Name(cluster=w1, "Image_Plugin_Data"=w3) -> (w2:T6)
  n14 = Build Array("") -> (w20:string[])
  n15 = node(w50, w30, w21, w9, w1, w2, w56, w20) -> (→"session out":refnum<k35>, w16:errorcluster, w28:T6, w17:string[])  [unwired: 2 in, 2 out]
  n16 = Delete From Array(array=w17) -> (deleted portion=w18:string)  [unwired: 2 in, 1 out]
  n17 = Search and Replace String(input string=w24, search string="Image") -> (result string=w5:string)  [unwired: 6 in, 3 out]
  n18 = Merge Errors(w16, w7) -> (w8:errorcluster)
  n19 = call "Remove Invisible Characters from String.vi"("String"=w5) -> ("result string"=w6:string)  [unwired: 3 in]
  n20 = call "AlliGator Get Message & Parameters from JSON Output.vi"("error in (no error)"=w8, "Function Display Name"=w11, "<JSON>"=w18) -> ("error out"=w15:errorcluster, "Notebook Message"=w12:string)  [unwired: 7 in]
  n21 = To Upper Case(1:w6) -> (0:w4:string)
  n22 = in-place {
    in-place-border: [w68] -> w59
    in-place-border: [w67] -> w36
    in-place-border: w28 -> [w66]
    in-place-border: w4 -> [w65]
    in-place-border: w21 -> [w61]
    in-place-border: w15 -> [w60]
    n23 = in-place-dvr #1("Data Value Reference in") -> (w63:T15)  [unwired: 1 out]
    n24 = Unbundle By Name(w66) -> ("Image_Plugin_Data.Image"=w64:sgl[][])
    n25 = case shown="Default" w65 {
      tunnel: w64 -> [_ w79 w90 w101 w112 w124]
      tunnel: [w72 w78 w89 w100 w111 w123] -> w68
      tunnel: [_ AlliGator_Variables_List."Phasor Plot:FLI Dataset Modified since last Calculation" ("Alligator Variable") AlliGator_Variables_List."Phasor Plot:FLI Dataset Modified since last Calculation" ("Alligator Variable") AlliGator_Variables_List."Phasor Plot:FLI Dataset Modified since last Calculation" AlliGator_Variables_List."Source Image:Mask Image Modified" ("Alligator Variable") AlliGator_Variables_List."Source Image:White Light Image Modified" ("Alligator Variable")] -> w67
      tunnel: w63 -> [w73 w76 w87 w98 w109 w121]
      tunnel: [w73 w75 w86 w97 w108 w120] -> w62
      tunnel: w61 -> [w71 _ _ _ _ _]
      tunnel: w60 -> [w69 w74 w85 w96 w107 w119]
      frame Default {
        n26 = call "AlliGator Check Invalid Python Plugin Output Value Type.vi"("error in (no error)"=w69, "Valid Output Value Type?"=FALSE, "Source"=w71) -> ("error out"=w72:errorcluster)  [unwired: 8 in]
      }
      frame "MAX" {
        n27 = in-place {
          in-place-border: w79 -> [w83]
          in-place-border: w74 -> [w81]
          in-place-border: [w82] -> w78
          n28 = in-place-cluster #2(w76) -> ("Current Dataset Images 1.SGL Max Image"=w80:T5)
          n29 = call "IMAQ ArrayToImage"("Image Pixels (Float)"=w83, "error in (no error)"=w81, "Image"=w80) -> ("error out"=w82:errorcluster, "Image Out"=w84:T5)  [unwired: 7 in]
          n30 = in-place-cluster #2("Current Dataset Images 1.SGL Max Image"=w84) -> (w75:T15)
        }
      }
      frame "MIN" {
        n31 = in-place {
          in-place-border: w90 -> [w94]
          in-place-border: w85 -> [w92]
          in-place-border: [w93] -> w89
          n32 = in-place-cluster #3(w87) -> ("Current Dataset Images 1.SGL Min Image"=w91:T5)
          n33 = call "IMAQ ArrayToImage"("Image Pixels (Float)"=w94, "error in (no error)"=w92, "Image"=w91) -> ("error out"=w93:errorcluster, "Image Out"=w95:T5)  [unwired: 7 in]
          n34 = in-place-cluster #3("Current Dataset Images 1.SGL Min Image"=w95) -> (w86:T15)
        }
      }
      frame "SUM" {
        n35 = in-place {
          in-place-border: w101 -> [w105]
          in-place-border: [w104] -> w100
          in-place-border: w96 -> [w103]
          n36 = in-place-cluster #4(w98) -> ("Current Dataset Images 1.SGL Sum Image"=w102:T5)
          n37 = call "IMAQ ArrayToImage"("Image Pixels (Float)"=w105, "error in (no error)"=w103, "Image"=w102) -> ("error out"=w104:errorcluster, "Image Out"=w106:T5)  [unwired: 7 in]
          n38 = in-place-cluster #4("Current Dataset Images 1.SGL Sum Image"=w106) -> (w97:T15)
        }
      }
      frame "MASK" {
        n39 = in-place {
          in-place-border: w112 -> [w118]
          in-place-border: [w116] -> w111
          in-place-border: w107 -> [w114]
          n40 = in-place-cluster #5(w109) -> ("Mask Image"=w113:T5)
          n41 = To Unsigned Word Integer(number=w118) -> (unsigned 16bit integer=w115:u16[][])
          n42 = call "IMAQ ArrayToImage"("Image Pixels (U16)"=w115, "error in (no error)"=w114, "Image"=w113) -> ("error out"=w116:errorcluster, "Image Out"=w117:T5)  [unwired: 7 in]
          n43 = in-place-cluster #5("Mask Image"=w117) -> (w108:T15)
        }
      }
      frame "WHITELIGHT" {
        n44 = in-place {
          in-place-border: w124 -> [w129]
          in-place-border: [w128] -> w123
          in-place-border: w119 -> [w127]
          n45 = in-place-cluster #6(w121) -> ("White Light Image"=w125:T5)
          n46 = To Unsigned Word Integer(number=w129) -> (unsigned 16bit integer=w126:u16[][])
          n47 = call "IMAQ ArrayToImage"("Image Pixels (U16)"=w126, "error in (no error)"=w127, "Image"=w125) -> ("error out"=w128:errorcluster, "Image Out"=w130:T5)  [unwired: 7 in]
          n48 = in-place-cluster #6("White Light Image"=w130) -> (w120:T15)
        }
      }
    }
    n49 = in-place-dvr #1(w62) -> (→"Data Value Reference out":refnum<data-value>)  [unwired: 1 out]
  }
  n50 = Format Into String(format string=" plugin:\n%s (%s)", initial string=w11, error in=w59, w12, w42) -> (resulting string=w40:string, error out=w39:errorcluster)
  n51 = Format Into String(format string=" used as %s", initial string=w40, error in=w39, w24) -> (resulting string=→"Message":string, error out=w38:errorcluster)
  n52 = call "Alligator Variables Storage.vi"("Get(F)/Set"=w35, "AlliGator Variable"=w36, "Error In"=w38, "Data in"=w35) -> ("Error Out"=→"error out":errorcluster)  [unwired: 5 in, 2 out]
